vi "op-run.vi"(0 "Chain IN":bool, 5 "Left Drive":dbl, 7 "Right Drive":dbl, 9 "Arm":dbl, 11 "Manipulator Position":dbl, 12 "Flag":bool, 13 "Arm Release":bool, 14 "Auto Servo":bool) -> (4 "Chain OUT":bool)   [LabVIEW 2010, in "LASA Beta.lvrbt"]
uses:
  LASA Beta.lvrbt
  <vilib>/NXT/NXTIO Xnodes/AddressXNode/NXTIOAddress.xnode
  <vilib>/NXT/Subs/MotorXNode.Servo Type.ctl
  <vilib>/NXT/Subs/MotorXNode.1Servo.ctl
  <vilib>/NXT/Subs/MotorXNode.3Servo.ctl
  <vilib>/NXT/Subs/MotorXNode.DC Motor Type.ctl
  <vilib>/NXT/Subs/MotorXNode.2DCMotor.ctl
  <vilib>/NXT/Subs/LVHSConnector.ctl
  <vilib>/NXT/NXTIO Xnodes/NXTIOXNode/NXTIO.xnode
  <vilib>/NXT/NXTIO Xnodes/NXTIONodeSubVIs/TETRIX IO Move Servos.vi
  <vilib>/NXT/NXTIO Xnodes/NXTIONodeSubVIs/TETRIX IO Move DC Motors.vi
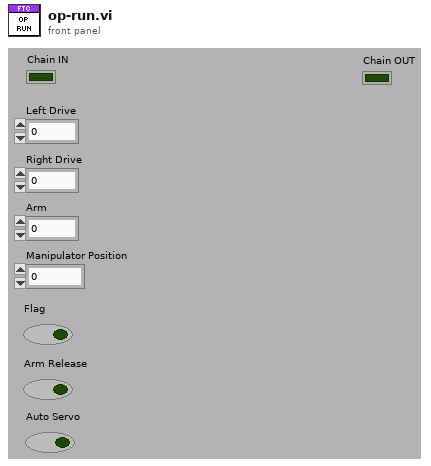
[diagram p1: front panel]
types:
  T1 = typedef "MotorXNode.DC Motor Type.ctl" = enum16{"DC Motor"}
  T2 = cluster{"DC Motor":T1, "Address":i16, "Address":i16}
  T3 = typedef "MotorXNode.Servo Type.ctl" = enum16{"Servo"}
  T4 = cluster{"Servo":T3, "Address":i16, "Address":i16, "Address":i16}
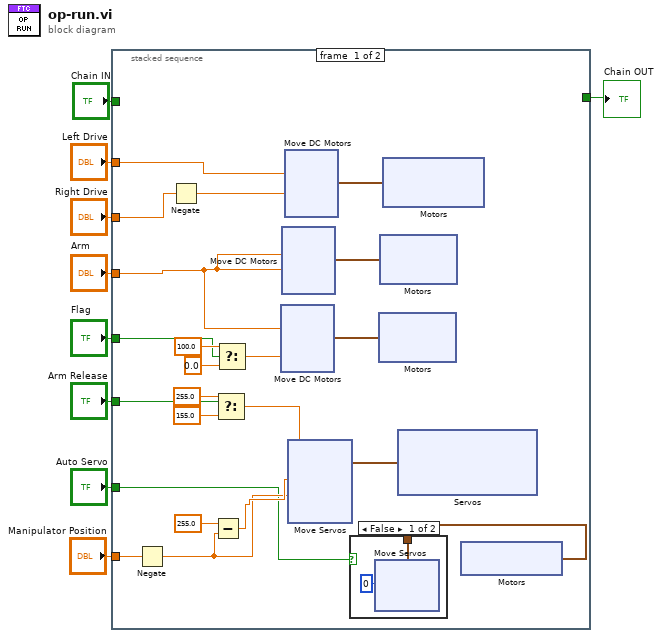
[diagram p0: block diagram]
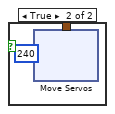
[diagram p2: hidden frame]
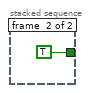
[diagram p3: hidden frame]
diagram:
  n1 = stacked-sequence {
    tunnel: "Chain IN" -> [_ _]
    tunnel: [_ TRUE] -> w8
    tunnel: "Left Drive" -> [w30 _]
    tunnel: "Right Drive" -> [w29 _]
    tunnel: "Arm" -> [w14 _]
    tunnel: "Flag" -> [w18 _]
    tunnel: "Arm Release" -> [w21 _]
    tunnel: "Auto Servo" -> [w11 _]
    tunnel: "Manipulator Position" -> [w16 _]
    frame #0 {
      n2 = Negate(x=w16) -> (-x=w13:dbl)
      n3 = Negate(x=w29) -> (-x=w28:dbl)
      n4 = Subtract(x=255.0, y=w13) -> (x-y=w15:dbl)
      n5 = Select(t=255.0, s=w21, f=155.0) -> (s? t:f=w10:dbl)
      n6 = Select(t=100.0, s=w18, f=0.0) -> (s? t:f=w23:dbl)
      n7 = xnode "Motors"() -> ("DC Motor"=w26:T2)
      n8 = xnode "Move DC Motors"("Power/Speed 2"=w23, "Power/Speed 1"=w14, "Motors"=w26) -> ()  [unwired: 1 in, 1 out]
      n9 = xnode "Motors"() -> ("DC Motor"=w27:T2)
      n10 = xnode "Move DC Motors"("Power/Speed 2"=w14, "Power/Speed 1"=w14, "Motors"=w27) -> ()  [unwired: 1 in, 1 out]
      n11 = xnode "Motors"() -> ("DC Motor"=w31:T2)
      n12 = xnode "Move DC Motors"("Power/Speed 2"=w28, "Power/Speed 1"=w30, "Motors"=w31) -> ()  [unwired: 1 in, 1 out]
      n13 = xnode "Servos"() -> ("Servo"=w22:T4)
      n14 = xnode "Move Servos"("Position 3"=w13, "Position 2"=w15, "Position 1"=w10, "Servos"=w22) -> ()  [unwired: 1 in, 1 out]
      n15 = xnode "Motors"() -> ("Servo"=w12:cluster{"Servo":T3, "Address":i16})
      n16 = case shown="False" w11 {
        tunnel: w12 -> [w33 w43]
        frame False {
          n17 = xnode "Move Servos"("Position 1"=u8 0, "Servos"=w33) -> ()  [unwired: 1 in, 1 out]
        }
        frame True {
          n18 = xnode "Move Servos"("Position 1"=u8 240, "Servos"=w43) -> ()  [unwired: 1 in, 1 out]
        }
      }
    }
    frame #1 {
    }
  }
  "Chain OUT" <- w8
